vi "貪食蛇_02_6_14.vi"(10 "reset":bool) -> (2 "®É¶¡(¬í)":dbl)   [LabVIEW 2014]
panel:
  out "Array":dbl[](array[numeric])
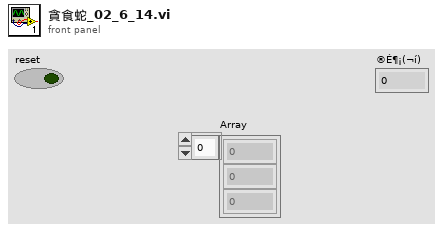
[diagram p1: front panel]
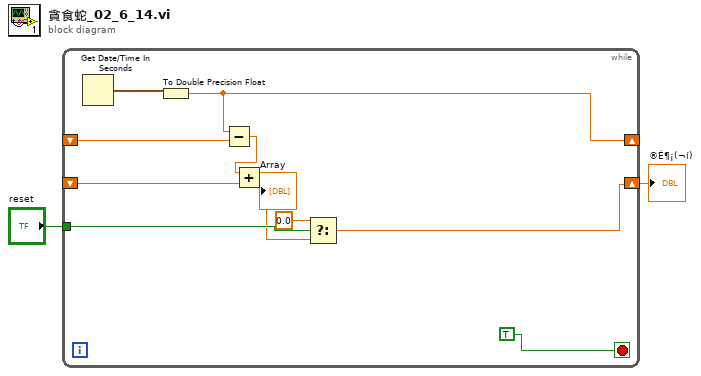
[diagram p0: block diagram]
diagram:
  n1 = while {
    shift-right: [w4] -> _
    shift-left: _ -> [w11]
    shift-right: [w5] -> w2
    shift-left: _ -> [w9]
    tunnel: "reset" -> [w8]
    stop <- TRUE stop-if-true
    n2 = Get Date/Time In Seconds() -> (seconds since 1Jan1904=w12:timestamp)
    n3 = To Double Precision Float(number=w12) -> (double precision float=w4:dbl)
    n4 = Subtract(x=w4, y=w11) -> (x-y=w10:dbl)
    n5 = Add(x=w10, y=w9) -> (x+y=w6:dbl)
    n6 = Select(t=0.0, s=w8, f=w6) -> (s? t:f=w5:dbl)
  }
  "®É¶¡(¬í)" <- w2
